vi "Arm Motor for shoot.vi"(1 "Motor input":dbl=-1.0, 2 "Current angle (deg)":dbl=133.60268690400002 format="%#_3g") -> ()   [LabVIEW 2013]
uses:
  <vilib>/Rock Robotics/WPI/RobotDrive/WPI_RobotDriveGetSetRefNum.vi
panel:
  out "Motor Output":T1(graph)={-100.0, "Current angle (deg)"=-1.0, "Angle"=150.04049090400002}
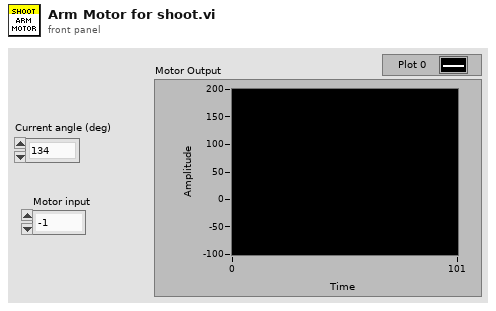
[diagram p1: front panel]
types:
  T1 = cluster{dbl, "Current angle (deg)":dbl, "Angle":dbl}
  T2 = typedef "WPI_RobotDriveDevRef.ctl" = cluster{"DevStatus":errorcluster, "Motors[]":T3[], "Square Inputs":bool, "Max Output":dbl, "Isochronous":bool}
  T3 = typedef "WPI_MotorControlDeviceRef.ctl" = cluster{"DeviceStatus":errorcluster, "Type":enum16{"PWM", "CAN"}, "PWM":cluster{"Digital Module":T4, "PWM Channel":T5, "DeadBand":T6}, "CAN":cluster{"Device Number":u8, "Control Mode":T7, "Semaphore":T8, "Max Vout":dbl}, "Invert":bool, "TransformRef":T9, "InvTransformRef":T9}
  T4 = typedef "FPGA_TypedefDigitalModule.ctl" = enum16{"Digital Module 1", "Digital Module 2"}
  T5 = typedef "FPGA_DIOPWMChannel.ctl" = enum8{"PWM 1", "PWM 2", "PWM 3", "PWM 4", "PWM 5", "PWM 6", "PWM 7", "PWM 8", "PWM 9", "PWM 10", "Invalid"}
  T6 = typedef "WPI_PWMDeadband.ctl" = cluster{"Name":string, "maxPositivePwm":i32, "minPositivePwm":i32, "centerPwm":i32, "maxNegativePwm":i32, "minNegativePwm":i32, "angularRange":u16}
  T7 = typedef "WPI_CANJaguar_ControlMode.ctl" = enum8{"Percent VBus", "Current", "Speed", "Position", "Voltage"}
  T8 = typedef "Semaphore RefNum" = refnum<k1>
  T9 = typedef "WPI_PWMTransform_ConPane.ctl" = refnum<vi>
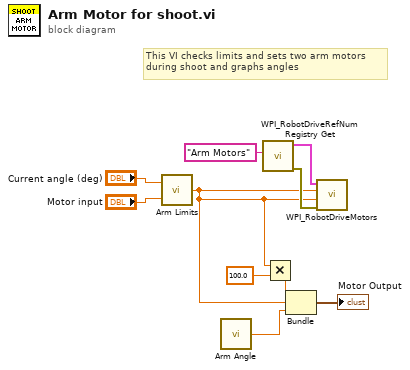
[diagram p0: block diagram]
diagram:
  # "This VI checks limits and sets two arm motors\nduring shoot and graphs angles"
  n1 = call "Arm Limits.vi"("Motor Input"="Motor input", "Current Angle"="Current angle (deg)") -> ("Motor Output"=w1:dbl)
  n2 = call "Arm Angle.vi"() -> ("Angle"=w3:dbl)  [unwired: 1 in, 2 out]
  n3 = call <vilib>:"WPI_RobotDriveRefNum Registry Get.vi"("refnum name"="Arm Motors") -> ("error out"=w7:errorcluster, "RobotDriveDevRef"=w8:T2)  [unwired: 9 in]
  n4 = Multiply(x=w1, y=100.0) -> (x*y=w5:dbl)
  n5 = Bundle(w5, "Motor Output"=w1, "Angle"=w3) -> (→"Motor Output":cluster{dbl, "Motor Output":dbl, "Angle":dbl})  [unwired: 1 in]
  n6 = call <vilib>:"WPI_RobotDriveMotors.vi"("error in (no error)"=w7, "RightSpeed"=w1, "LeftSpeed"=w1, "RobotDriveDevRef"=w8) -> ()  [unwired: 5 in, 3 out]
